vi "Main.vi"() -> ()   [LabVIEW 2017, in "Akwizycja.lvlib"]
doc: "This template is based from the Queued Message Handler design pattern and the Queued Message Handler Project Template that ships with LabVIEW 2014.\n\nThe main difference is that the Queue is private to this module and communication between modules is done via Broadcast and Request events.\n\nRequest events are wrapped via public API methods and are handled in the Event handler loop in this VI.\nAny module can register for Broadcast events sent by this module.\n\nThe Event Handling Loop generates messages based on user interface actions.\n\nThe Message Handling Loop processes messages generated by the Event Handling Loop, or by other messages. The messages are string values, so new messages can be added easily to the Message Cases case structure in the Message Handling Loop. Each message cluster can also provide an optional value for Message Data, which is a variant that can be converted to whatever message-specific data is required.\n_____\nBased on Delacor QMH Project Template 3.1.0.34."
uses:
  Akwizycja.lvlib
  <vilib>/Delacor/Delacor QMH/Libraries/Module Admin_class/Delacor_lib_QMH_Module Admin.lvclass
  Time Events cluster.ctl
  Time events enum.ctl
  Module Data--cluster.ctl
  Show Panel Argument--cluster.ctl
  Hide Panel Argument--cluster.ctl
  Stop Argument--cluster.ctl
  <vilib>/Delacor/Delacor QMH/Libraries/Module Admin_class/Delacor_lib_QMH_Module Admin.lvclass/Delacor_lib_QMH_Module Admin.ctl
  Read Slaves Argument--cluster.ctl
  <vilib>/Utility/miscctls.llb/LVPointTypeDef.ctl
  <vilib>/Delacor/Delacor QMH/Libraries/Module Admin_class/Delacor_lib_QMH_Get External Launch.vi
  <vilib>/Utility/error.llb/Error Cluster From Error Code.vi
  <vilib>/Delacor/Delacor QMH/Libraries/Message Queue_class/Delacor_lib_QMH_Enqueue Message (Single).vi
  <vilib>/ErrorRing/Error Ring.xnode
  <vilib>/Delacor/Delacor QMH/Libraries/Message Queue_class/Delacor_lib_QMH_Message Queue.lvclass
  <vilib>/Plasmionique/MB Master/MB_Master_Serial/MB_Master_Serial.lvclass
panel:
  out "error obsrany":errorcluster
  in  "log_avg_c":dbl
  in  "Time Events":T1
  in  "Registers 2":u16[][](array[numeric])
  out "read_slaves":bool
  out "Elapsed Time (s)":dbl
  out "stop_time":bool
  in  "Simulate MHL Error":bool
  in  "Simulate EHL Error":bool
  out "error out":errorcluster
  in  "Module Admin":refnum<class "Delacor_lib_QMH_Module Admin.lvclass">
  out "Status":string
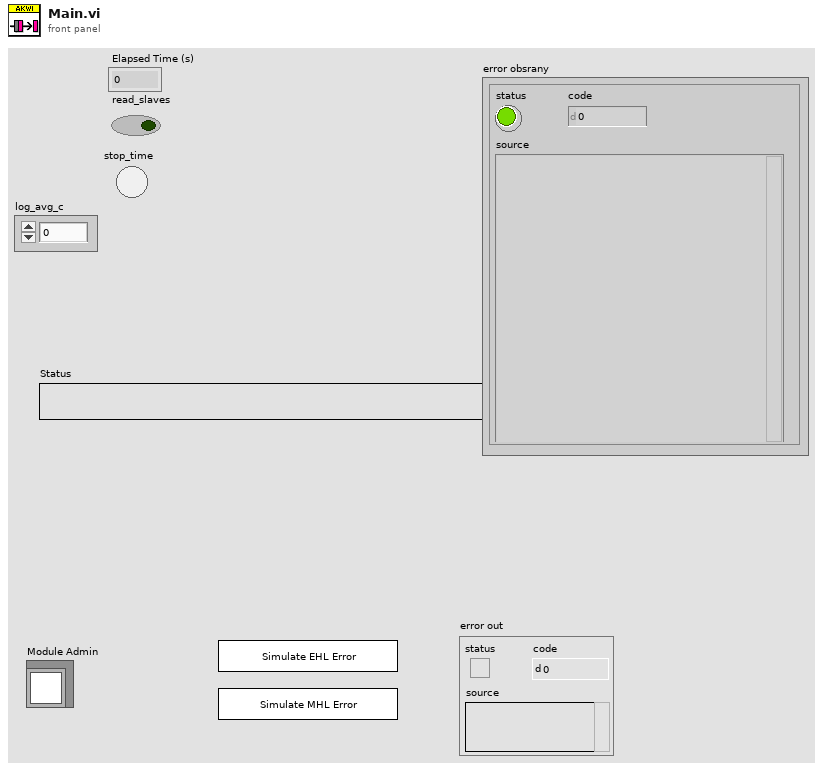
[diagram p1: front panel]
types:
  T1 = typedef "Time Events cluster.ctl" = cluster{"Read Slaves":refnum<user-event>, "Log Avg":refnum<user-event>}
  T2 = typedef "Time events enum.ctl" = enum16{"read_slaves", "log_avg"}
  T3 = typedef "Akwizycja.lvlib/Request Events--cluster.ctl" = cluster{"Stop Module":refnum<user-event>, "Show Panel":refnum<user-event>, "Hide Panel":refnum<user-event>, "Get Module Execution Status":refnum<user-event>, "Show Diagram":refnum<user-event>, "Read Slaves":refnum<user-event>}
  T4 = typedef "Akwizycja.lvlib/Module Data--cluster.ctl" = cluster{"Status":string}
  T5 = typedef "Akwizycja.lvlib/Show Panel Argument--cluster.ctl" = cluster{"Show Panel?":bool}
  T6 = typedef "Akwizycja.lvlib/Hide Panel Argument--cluster.ctl" = cluster{"Hide Panel?":bool}
  T7 = typedef "Akwizycja.lvlib/Stop Argument--cluster.ctl" = cluster{"Origin":string, "Exit via Stop Module Req?":bool, "Wait for Module to stop?":bool}
  T8 = typedef "Akwizycja.lvlib/Read Slaves Argument--cluster.ctl" = cluster{"Boolean":bool}
  T9 = typedef "LVPointTypeDef.ctl" = cluster{"Horizontal":i16, "Vertical":i16}
  T10 = enum32{"Invalid", "Standard", "Closed", "Hidden", "Minimized", "Maximized"}
  T11 = enum32{"invalid lock state", "Not Locked", "Locked (No Password)", "Password-protected"}
  T12 = cluster{"Fuel Flow":dbl[][][], "Init array":refnum<class "MB_Master_Serial.lvclass">[], "Array of temperatures":dbl[][][]}
  T13 = cluster{"Fuel Flow":dbl[][][], "Init array":refnum<class "MB_Master_Serial.lvclass">[], "Temps":dbl[][][]}
  T14 = cluster{"Combined Fuel Flows":dbl[][][], "Serial out":refnum<class "MB_Master_Serial.lvclass">[], "Combined Temps":dbl[][][]}
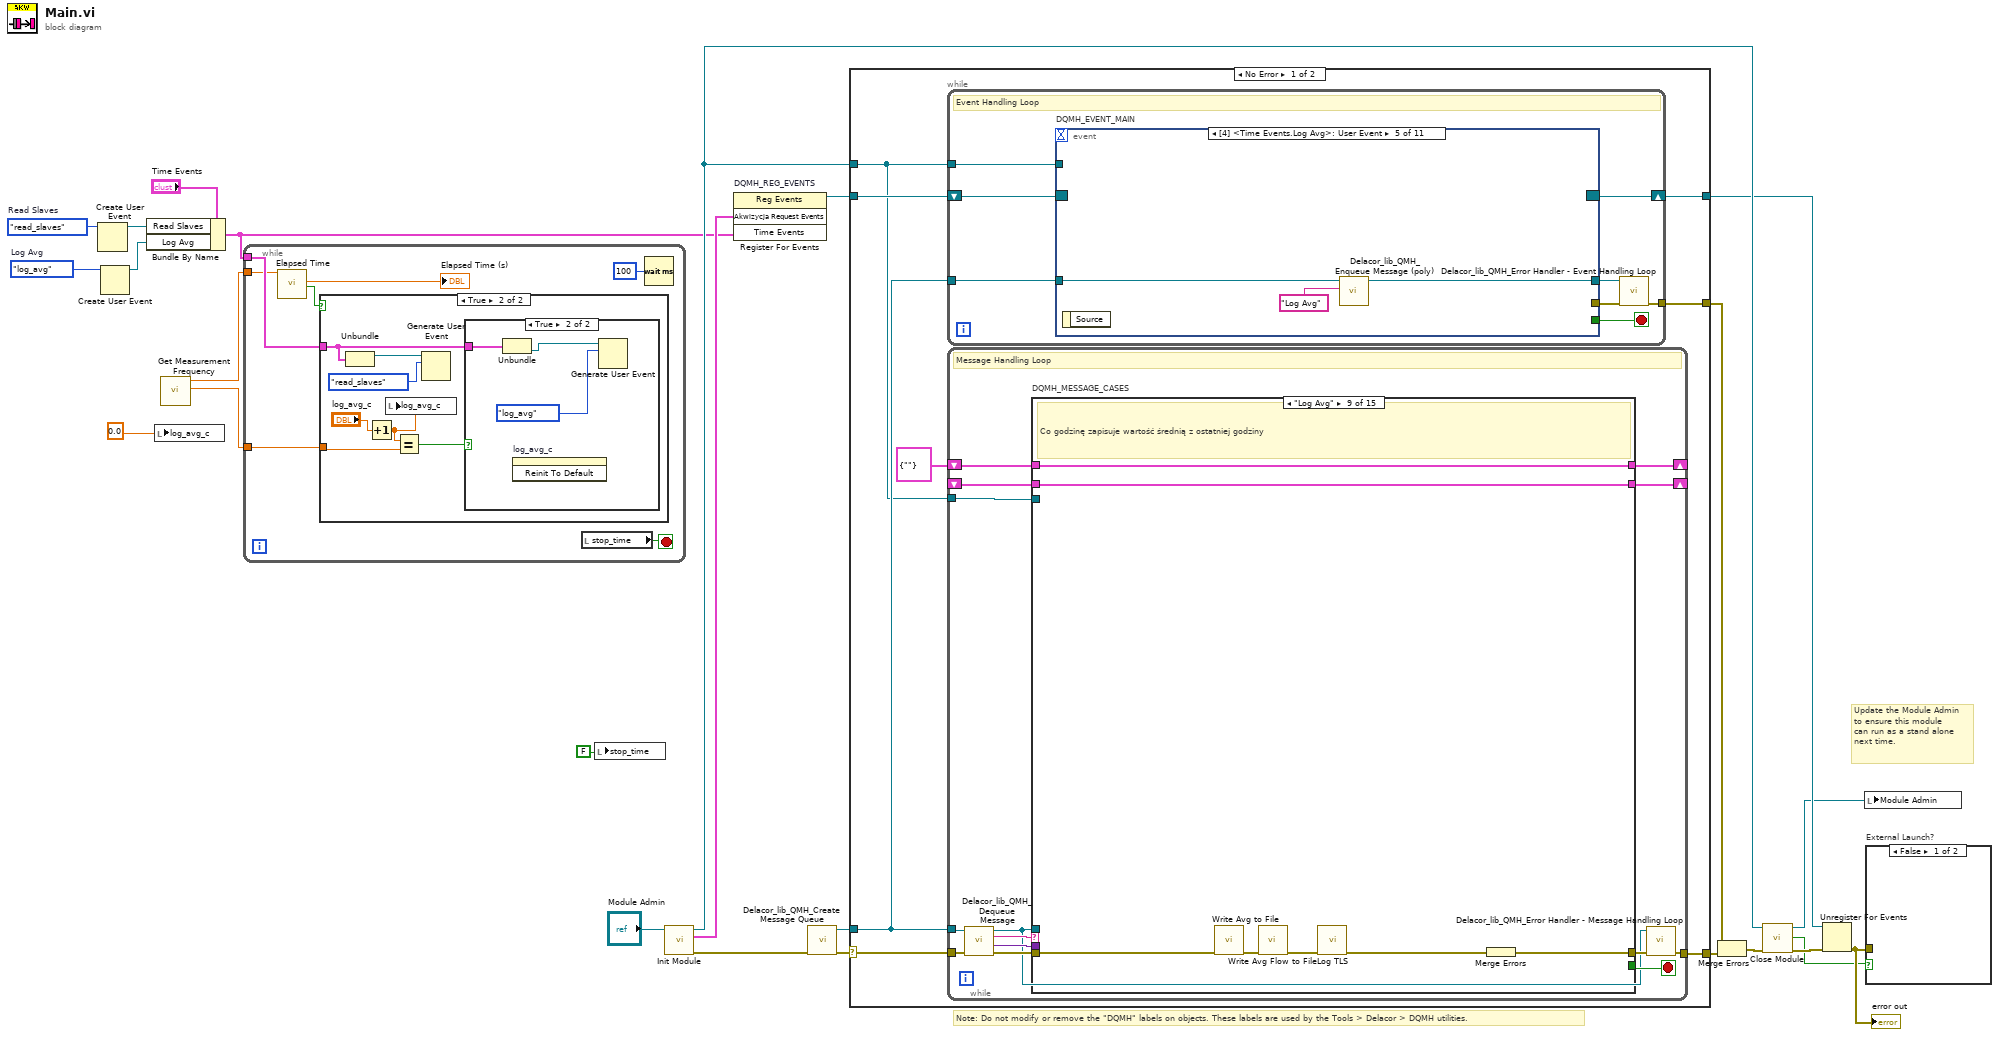
[diagram p0: block diagram]
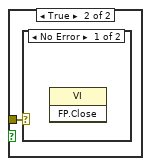
[diagram p4: hidden frame]
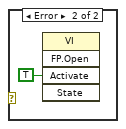
[diagram p5: hidden frame]
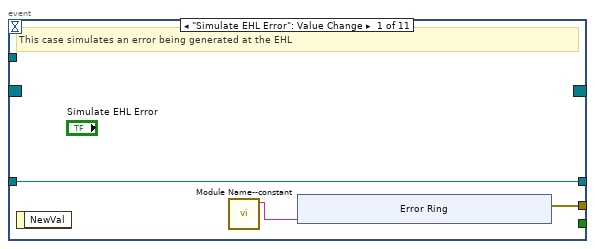
[diagram p6: hidden frame]
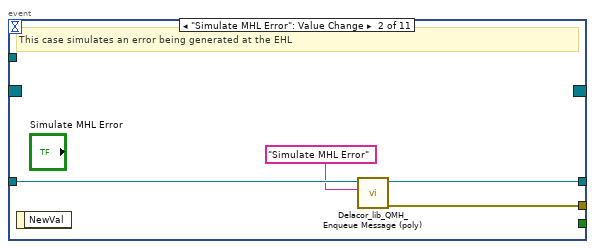
[diagram p7: hidden frame]
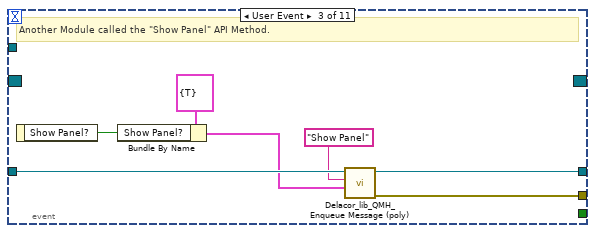
[diagram p8: hidden frame]
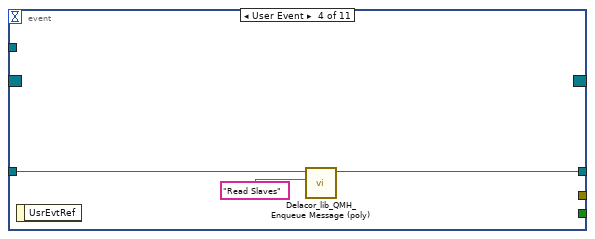
[diagram p9: hidden frame]
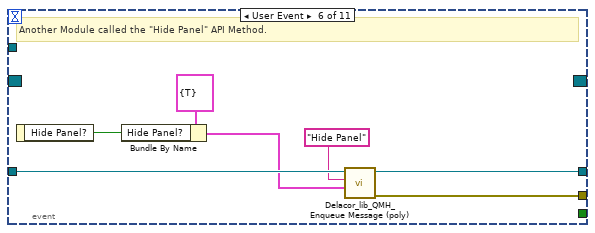
[diagram p10: hidden frame]
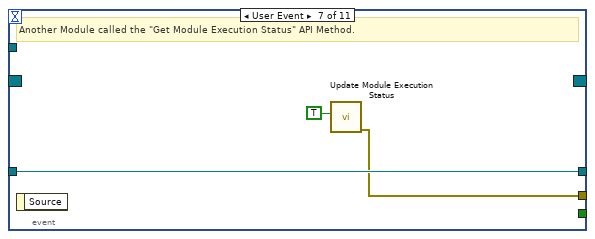
[diagram p11: hidden frame]
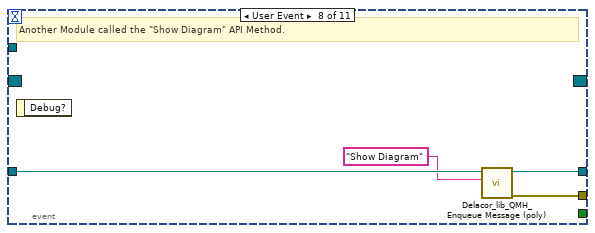
[diagram p12: hidden frame]
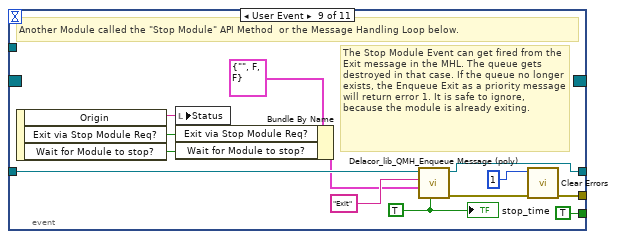
[diagram p13: hidden frame]
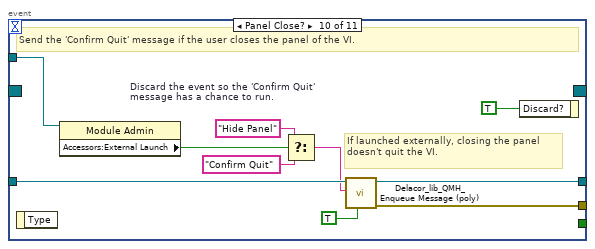
[diagram p14: hidden frame]
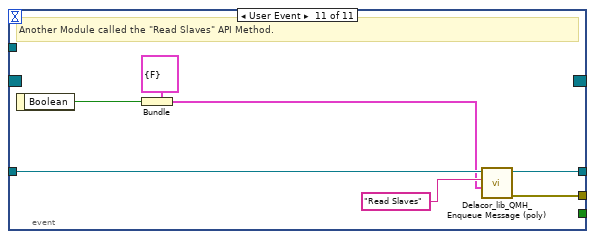
[diagram p15: hidden frame]
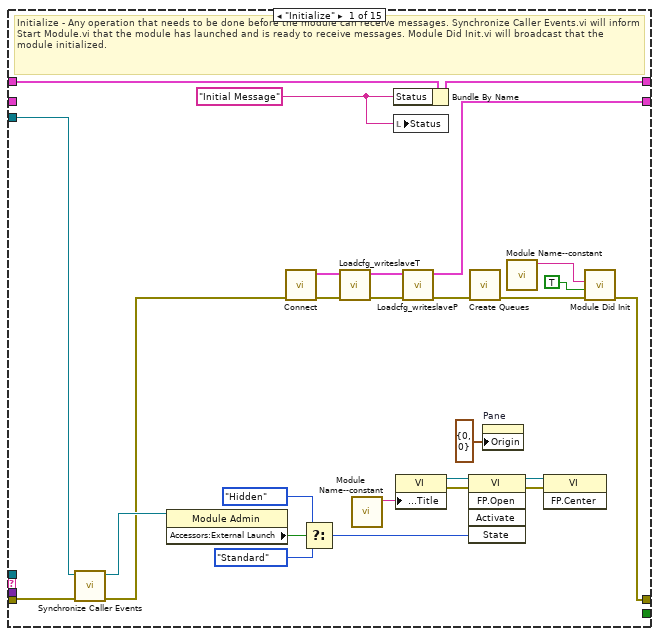
[diagram p16: hidden frame]
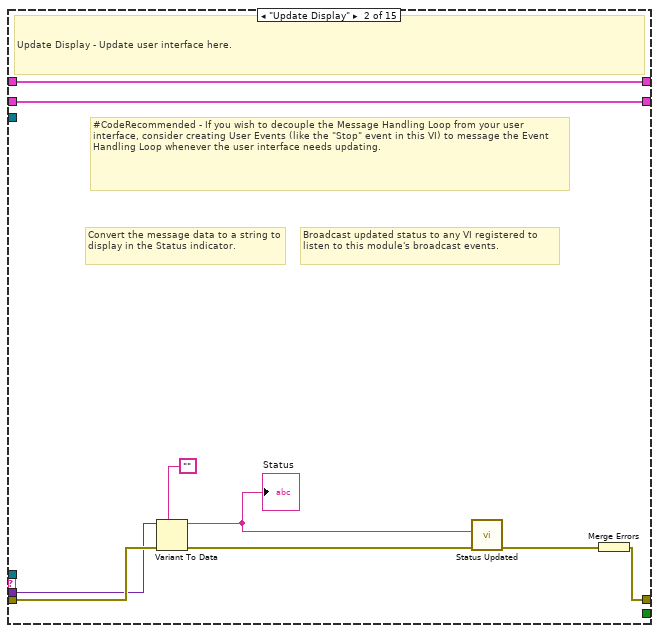
[diagram p17: hidden frame]
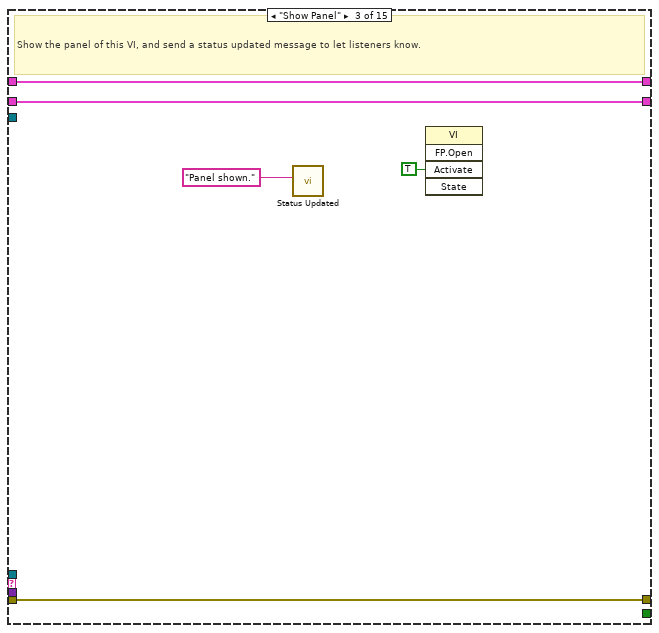
[diagram p18: hidden frame]
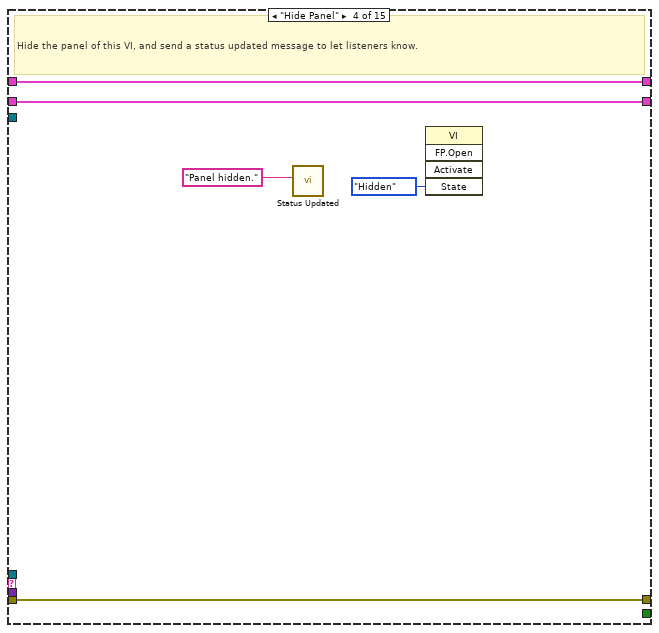
[diagram p19: hidden frame]
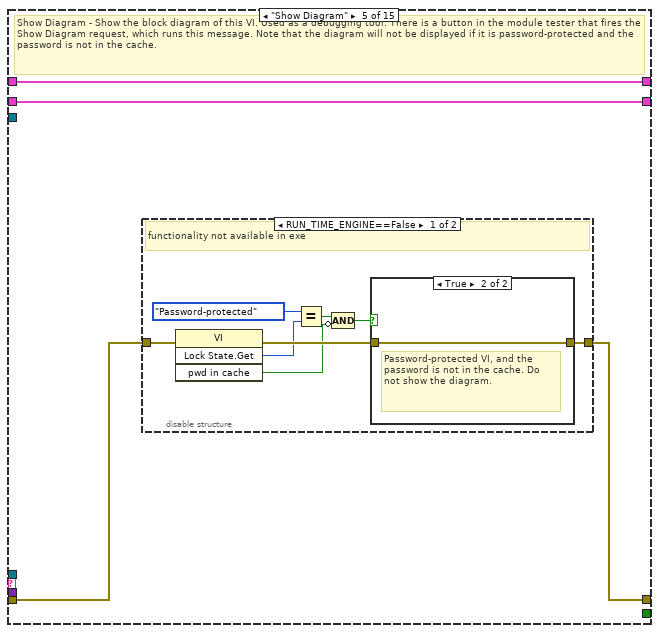
[diagram p20: hidden frame]
diagram:
  w5 = Time_events_enum."log_avg"  # Log Avg
  w9 = Time_events_enum."read_slaves"  # Read Slaves
  # "Note: Do not modify or remove the \"DQMH\" labels on objects. These labels are used by the Tools > Delacor > DQMH utilities."
  # "Update the Module Admin to ensure this module can run as a stand alone next time."
  n1 = Create User Event(user event datatype=w9) -> (user event=w8:refnum<user-event>)  [unwired: 1 in, 1 out]
  n2 = Create User Event(user event datatype=w5) -> (user event=w4:refnum<user-event>)  [unwired: 1 in, 1 out]
  n3 = Bundle By Name(cluster="Time Events", "Read Slaves"=w8, "Log Avg"=w4) -> (w6:T1)
  n4 = local write "log_avg_c"(0.0 ("log_avg_c")) -> ()
  n5 = call "Get Measurement Frequency.vi"() -> ("Measurments per hour"=w2:dbl, "Seconds"=w3:dbl)  [unwired: 10 in]
  n6 = while {
    tunnel: w6 -> [w28]
    tunnel: w3 -> [w27]
    tunnel: w2 -> [w26]
    stop <- w30 stop-if-true
    n7 = call "Elapsed Time"("Time Target (s)"=w27) -> ("Elapsed Time (s)"=→"Elapsed Time (s)":dbl, "Time has Elapsed"=w29:bool)  [unwired: 11 in, 6 out]
    n8 = case shown="True" w29 {
      tunnel: w28 -> [_ w33]
      tunnel: w26 -> [_ w35]
      frame False {
      }
      frame True {
        n9 = Unbundle(w33) -> ("Read Slaves"=w38:refnum<user-event>)  [unwired: 1 out]
        n10 = Increment(x="log_avg_c") -> (x+1=w36:dbl)
        n11 = local write "log_avg_c"(w36) -> ()
        n12 = Equal?(x=w36, y=w35) -> (x = y?=w34:bool)
        n13 = Generate User Event(user event=w38, event data cluster=Time_events_enum."read_slaves") -> ()  [unwired: 2 in, 2 out]
        n14 = case shown="True" w34 {
          tunnel: w33 -> [_ w40]
          frame False {
          }
          frame True {
            n15 = Unbundle(w40) -> ("Log Avg"=w41:refnum<user-event>)  [unwired: 1 out]
            n16 = invoke on="log_avg_c" class="DigNum (strict)" method="Reinit To Default"() -> ()  [unwired: 3 in, 3 out]
            n17 = Generate User Event(user event=w41, event data cluster=Time_events_enum."log_avg") -> ()  [unwired: 2 in, 2 out]
          }
        }
      }
    }
    n18 = local read "stop_time"() -> (w30:bool)
    n19 = Wait (ms)(milliseconds to wait=u32 100) -> ()  [unwired: 1 out]
  }
  n20 = local write "stop_time"(FALSE) -> ()
  n21 = call "Init Module.vi"("Singleton Module Admin in"="Module Admin") -> ("error out"=w23:errorcluster, "Akwizycja Request Events"=w20:T3, "Singleton Module Admin out"=w25:refnum<class "Delacor_lib_QMH_Module Admin.lvclass">)  [unwired: 8 in]
  n22 = register-events "DQMH_REG_EVENTS"(w20, w6) -> (reference out=w21:refnum<event-registration>)  [unwired: 2 in, 1 out]
  n23 = call <vilib>:"Delacor_lib_QMH_Create Message Queue.vi"("error in (no error)"=w23) -> ("error out"=w11:errorcluster, "Message Queue"=w19:refnum<class "Delacor_lib_QMH_Message Queue.lvclass">)  [unwired: 9 in]
  n24 = case shown="No Error" w11 {
    selector: w11 -> [w44 w378]
    tunnel: [w50 w378] -> w24
    tunnel: [w49 w383] -> w22
    tunnel: w21 -> [w47 w383]
    tunnel: w19 -> [w46 _]
    tunnel: [w45 _] -> w15
    tunnel: w25 -> [w43 w379]
    frame No Error {
      n25 = while {
        tunnel: w46 -> [w58]
        shift-right: [w56] -> w49
        shift-left: w47 -> [w57]
        tunnel: [w52] -> w45
        tunnel: w43 -> [w51]
        stop <- w54 stop-if-true
        # "Event Handling Loop"
        n26 = event "DQMH_EVENT_MAIN" shown="[4] <Time Events.Log Avg>: User Event" {
          selector: w57 -> [_ _ _ _ _ _ _ _ _ _ _]
          dyn-events: [_ _ _ _ _ _ _ _ _ _ _] -> w56
          timeout: _ -> [_ _ _ _ _ _ _ _ _ _ _]
          tunnel: [_ _ _ _ _ _ _ _ TRUE ("Discard?") _ _] -> w54
          tunnel: w58 -> [w61 w72 w79 w82 w84 w92 w95 w99 w110 w121 w129]
          tunnel: [w60 w69 w77 _ _ w90 w94 w96 w105 w120 w123] -> w55
          tunnel: [w61 w71 w78 w81 w83 w91 w95 w98 w109 w119 w128] -> w53
          tunnel: w51 -> [_ _ _ _ _ _ _ _ _ w115 _]
          event "Simulate EHL Error": Value Change {
            # "This case simulates an error being generated at the EHL"
            n27 = event-data() -> ()  [unwired: 1 in, 1 out]
            n28 = call "Module Name--constant.vi"() -> ("Module Name"=w59:string)  [unwired: 11 in]
            n29 = xnode "Error Ring"("parameter 0"=w59) -> ("error out"=w60:errorcluster)
          }
          event "Simulate MHL Error": Value Change {
            # "This case simulates an error being generated at the EHL"
            n30 = event-data() -> ()  [unwired: 1 in, 1 out]
            n31 = call-poly <vilib>:"Delacor_lib_QMH_Enqueue Message (poly).vi"("Message"="Simulate MHL Error", "Message Queue in"=w72) -> ("error out"=w69:errorcluster, "Message Queue out"=w71:refnum<class "Delacor_lib_QMH_Message Queue.lvclass">)  [unwired: 8 in]
          }
          event User Event {
            # "Another Module called the \"Show Panel\" API Method."
            n32 = event-data() -> ("Show Panel?"=w75:bool)  [unwired: 1 in]
            n33 = Bundle By Name(cluster=T5 {"Show Panel?"=TRUE} ("Show Panel Argument"), "Show Panel?"=w75) -> (w73:T5)
            n34 = call-poly <vilib>:"Delacor_lib_QMH_Enqueue Message (poly).vi"("Message Data"=w73, "Message"="Show Panel", "Message Queue in"=w79) -> ("error out"=w77:errorcluster, "Message Queue out"=w78:refnum<class "Delacor_lib_QMH_Message Queue.lvclass">)  [unwired: 7 in]
          }
          event User Event {
            n35 = event-data() -> ()  [unwired: 1 in, 1 out]
            n36 = call-poly <vilib>:"Delacor_lib_QMH_Enqueue Message (poly).vi"("Message"="Read Slaves", "Message Queue in"=w82) -> ("Message Queue out"=w81:refnum<class "Delacor_lib_QMH_Message Queue.lvclass">)  [unwired: 8 in, 1 out]
          }
          event User Event {
            n37 = event-data() -> ()  [unwired: 1 in, 1 out]
            n38 = call-poly <vilib>:"Delacor_lib_QMH_Enqueue Message (poly).vi"("Message"="Log Avg", "Message Queue in"=w84) -> ("Message Queue out"=w83:refnum<class "Delacor_lib_QMH_Message Queue.lvclass">)  [unwired: 8 in, 1 out]
          }
          event User Event {
            # "Another Module called the \"Hide Panel\" API Method."
            n39 = event-data() -> ("Hide Panel?"=w87:bool)  [unwired: 1 in]
            n40 = Bundle By Name(cluster=T6 {"Hide Panel?"=TRUE} ("Hide Panel Argument"), "Hide Panel?"=w87) -> (w86:T6)
            n41 = call-poly <vilib>:"Delacor_lib_QMH_Enqueue Message (poly).vi"("Message Data"=w86, "Message"="Hide Panel", "Message Queue in"=w92) -> ("error out"=w90:errorcluster, "Message Queue out"=w91:refnum<class "Delacor_lib_QMH_Message Queue.lvclass">)  [unwired: 7 in]
          }
          event User Event {
            # "Another Module called the \"Get Module Execution Status\" API Method."
            n42 = event-data() -> ()  [unwired: 1 in, 1 out]
            n43 = call "Update Module Execution Status.vi"("Running?"=TRUE) -> ("error out"=w94:errorcluster)  [unwired: 10 in]
          }
          event User Event {
            # "Another Module called the \"Show Diagram\" API Method."
            n44 = event-data() -> ()  [unwired: 1 in, 1 out]
            n45 = call-poly <vilib>:"Delacor_lib_QMH_Enqueue Message (poly).vi"("Message"="Show Diagram", "Message Queue in"=w99) -> ("error out"=w96:errorcluster, "Message Queue out"=w98:refnum<class "Delacor_lib_QMH_Message Queue.lvclass">)  [unwired: 8 in]
          }
          event User Event {
            w100 = TRUE ("Priority Message? (F)")
            # "The Stop Module Event can get fired from the Exit message in the MHL. The queue gets destroyed in that case. If the queue no longer exists, the Enqueue Exit as a priority message will return error 1. It is safe to ignore, because the module is already exiting."
            # "Another Module called the \"Stop Module\" API Method  or the Message Handling Loop below."
            n46 = event-data() -> ("Origin"=w108:string, "Exit via Stop Module Req?"=w103:bool, "Wait for Module to stop?"=w102:bool)  [unwired: 1 in]
            n47 = local write "Status"(w108) -> ()
            n48 = Bundle By Name(cluster=T7 {"Origin"="", "Exit via Stop Module Req?"=FALSE, "Wait for Module to stop?"=FALSE} ("Stop Argument"), "Exit via Stop Module Req?"=w103, "Wait for Module to stop?"=w102) -> (w101:T7)
            n49 = call-poly <vilib>:"Delacor_lib_QMH_Enqueue Message (poly).vi"("Priority Message? (F)"=w100, "Message Data"=w101, "Message"="Exit", "Message Queue in"=w110) -> ("error out"=w106:errorcluster, "Message Queue out"=w109:refnum<class "Delacor_lib_QMH_Message Queue.lvclass">)  [unwired: 6 in]
            n50 = call <vilib>:"Clear Errors.vi"("error in (no error)"=w106, "specific error code to clear (0: all)"=1) -> ("error out"=w105:errorcluster)  [unwired: 4 in, 1 out]
            "stop_time" <- w100
          }
          event Panel Close? {
            w122 = TRUE  # Discard the event so the 'Confirm Quit' message has a chance to run.
            # "If launched externally, closing the panel doesn't quit the VI."
            # "Send the 'Confirm Quit' message if the user closes the panel of the VI."
            n51 = event-data() -> ()  [unwired: 1 in, 1 out]
            n52 = property class="Module Admin"(reference=w115) -> ("Accessors:External Launch"=w114:bool)  [unwired: 1 in, 2 out]
            n53 = Select(t="Hide Panel" ("Message"), s=w114, f="Confirm Quit" ("Message")) -> (s? t:f=w116:string)
            n54 = call-poly <vilib>:"Delacor_lib_QMH_Enqueue Message (poly).vi"("Priority Message? (F)"=TRUE, "Message"=w116, "Message Queue in"=w121) -> ("error out"=w120:errorcluster, "Message Queue out"=w119:refnum<class "Delacor_lib_QMH_Message Queue.lvclass">)  [unwired: 7 in]
            n55 = event-data("Discard?"=w122) -> ()  [unwired: 1 in, 1 out]
          }
          event User Event {
            # "Another Module called the \"Read Slaves\" API Method."
            n56 = event-data() -> ("Boolean"=w124:bool)  [unwired: 1 in]
            n57 = Bundle(cluster=T8 {"Boolean"=FALSE} ("Read Slaves Argument"), "Boolean"=w124) -> (w125:T8)
            n58 = call-poly <vilib>:"Delacor_lib_QMH_Enqueue Message (poly).vi"("Message Data"=w125, "Message"="Read Slaves", "Message Queue in"=w129) -> ("error out"=w123:errorcluster, "Message Queue out"=w128:refnum<class "Delacor_lib_QMH_Message Queue.lvclass">)  [unwired: 7 in]
          }
        }
        n59 = call-dynamic "Delacor_lib_QMH_Error Handler - Event Handling Loop.vi"("error in (no error)"=w55, "Message Queue in"=w53) -> ("dup error in"=w52:errorcluster)  [unwired: 8 in, 1 out]
      }
      n60 = while {
        tunnel: w46 -> [w135]
        shift-right: [w141] -> _
        shift-left: T4 {"Status"=""} ("Data Cluster") -> [w142]
        tunnel: w44 -> [w139]
        tunnel: [w134] -> w50
        tunnel: w43 -> [w133]
        shift-right: [w132] -> _
        shift-left: _ -> [w131]
        stop <- w140 stop-if-true
        # "Message Handling Loop"
        n61 = call-dynamic "Delacor_lib_QMH_Dequeue Message.vi"("error in (no error)"=w139, "Message Queue in"=w135) -> ("error out"=w138:errorcluster, "Message Data"=w136:variant, "Message"=w137:string, "Message Queue out"=w130:refnum<class "Delacor_lib_QMH_Message Queue.lvclass">)  [unwired: 6 in]
        n62 = case "DQMH_MESSAGE_CASES" shown="\"Log Avg\"" w137 {
          selector: w137 -> [_ _ _ _ _ _ _ _ _ _ _ _ _ _ w365]
          tunnel: w130 -> [_ _ _ _ _ _ _ w239 _ _ _ w299 w331 w357 _]
          tunnel: w138 -> [w160 w177 w184 w186 w192 w208 w232 w238 w270 w277 w283 w303 w335 w359 _]
          tunnel: [w147 w178 w184 w186 w191 w214 w230 w241 w272 w275 w281 w294 w333 w354 w366] -> w143
          tunnel: w142 -> [w159 w179 w183 w189 w193 w228 w231 w242 w273 w276 w282 w302 w334 w356 w367]
          tunnel: [w158 w179 w183 w189 w193 w228 w231 w242 w273 w276 w282 w302 w334 w356 w367] -> w141
          tunnel: [_ _ _ _ _ _ _ _ _ _ _ _ _ w346 _] -> w140
          tunnel: w136 -> [_ w176 _ _ _ _ _ _ _ _ _ w301 _ w353 _]
          tunnel: w133 -> [w161 _ _ _ _ _ _ _ _ _ _ w298 _ w347 _]
          tunnel: [w144 w171 w180 w185 w190 w224 w229 w236 w271 w274 w278 w296 w328 w338 w363] -> w132
          tunnel: w131 -> [_ w171 w180 w185 w190 w225 w229 w240 w271 w274 w278 w296 w328 w338 w363]
          frame "Initialize" {
            w157 = "Initial Message" ("Initial Message")
            # "Initialize - Any operation that needs to be done before the module can receive messages. Synchronize Caller Events.vi will inform Start Module.vi that the module has launched and is ready to receive messages. Module Did Init.vi will broadcast that the module initialized."
            n63 = call "Synchronize Caller Events.vi"("error in (no error)"=w160, "Singleton Module Admin in"=w161) -> ("error out"=w148:errorcluster, "Singleton Module Admin out"=w156:refnum<class "Delacor_lib_QMH_Module Admin.lvclass">)  [unwired: 8 in]
            n64 = property class="Module Admin"(reference=w156) -> ("Accessors:External Launch"=w165:bool)  [unwired: 1 in, 2 out]
            n65 = call "Connect.vi"("error in"=w148) -> ("error out"=w153:errorcluster, "Data Cluster"=w146:T12)  [unwired: 9 in]
            n66 = Select(t=T10."Hidden" ("State"), s=w165, f=T10."Standard" ("State")) -> (s? t:f=w162:T10)
            n67 = call "Loadcfg_writeslaveT.vi"("error in"=w153, "Data Cluster in"=w146) -> ("error out"=w154:errorcluster, "Data Cluster out"=w145:T13)  [unwired: 8 in]
            n68 = call "Module Name--constant.vi"() -> ("Module Name"=w170:string)  [unwired: 11 in]
            n69 = Bundle By Name(cluster=w159, "Status"=w157) -> (w158:T4)
            n70 = local write "Status"(w157) -> ()
            n71 = property class="VI"("Front Panel.Title"=w170) -> (reference out=w168:refnum<vi>, error out=w169:errorcluster)  [unwired: 2 in]
            n72 = call "Loadcfg_writeslaveP.vi"("error in"=w154, "Data Cluster in"=w145) -> ("error out"=w150:errorcluster, "Data Cluster out"=w144:T13)  [unwired: 8 in]
            n73 = invoke class="VI" method="FP.Open"(reference=w168, error in=w169, "State"=w162) -> (reference out=w167:refnum<vi>, error out=w166:errorcluster)  [unwired: 2 in, 3 out]
            n74 = call "Create Queues.vi"("error in (no error)"=w150) -> ("error out"=w149:errorcluster)  [unwired: 10 in]
            n75 = property on="Pane" class="Pane"("Origin"=T9 {"Horizontal"=0, "Vertical"=0}) -> ()  [unwired: 2 in, 2 out]
            n76 = call "Module Name--constant.vi"() -> ("Module Name"=w152:string)  [unwired: 11 in]
            n77 = invoke class="VI" method="FP.Center"(reference=w167, error in=w166) -> ()  [unwired: 1 in, 3 out]
            n78 = call "Module Did Init.vi"("error in (no error)"=w149, "Initialized?"=TRUE, "Origin"=w152) -> ("error out"=w147:errorcluster)  [unwired: 8 in]
          }
          frame "Update Display" {
            # "Broadcast updated status to any VI registered to listen to this module's broadcast events."
            # "Convert the message data to a string to display in the Status indicator."
            # "#CodeRecommended - If you wish to decouple the Message Handling Loop from your user interface, consider creating User Events (like the \"Stop\" event in this VI) to message the Event Handling Loop whenever the user interface needs updating."
            # "Update Display - Update user interface here."
            n79 = Variant To Data(error in=w177, type="", Variant=w176) -> (data=w174:string, error out=w173:errorcluster)
            "Status" <- w174
            n80 = call "Status Updated.vi"("error in (no error)"=w173, "Status"=w174) -> ("error out"=w172:errorcluster)  [unwired: 9 in]
            n81 = Merge Errors(w172) -> (w178:errorcluster)
          }
          frame "Show Panel" {
            # "Show the panel of this VI, and send a status updated message to let listeners know."
            n82 = call "Status Updated.vi"("Status"="Panel shown." ("format string")) -> ()  [unwired: 10 in, 1 out]
            n83 = invoke class="VI" method="FP.Open"("Activate"=TRUE ("Activate?")) -> ()  [unwired: 4 in, 5 out]
          }
          frame "Hide Panel" {
            # "Hide the panel of this VI, and send a status updated message to let listeners know."
            n84 = call "Status Updated.vi"("Status"="Panel hidden." ("format string")) -> ()  [unwired: 10 in, 1 out]
            n85 = invoke class="VI" method="FP.Open"("State"=T10."Hidden") -> ()  [unwired: 4 in, 5 out]
          }
          frame "Show Diagram" {
            # "Show Diagram - Show the block diagram of this VI. Used as a debugging tool. There is a button in the module tester that fires the Show Diagram request, which runs this message. Note that the diagram will not be displayed if it is password-protected and the password is not in the cache."
            n86 = disable-structure shown="RUN_TIME_ENGINE==False" {
              disable-tunnel: [w201 w207] -> w191
              disable-tunnel: w192 -> [w200 w207]
              frame condition #0 (active) {
                # "functionality not available in exe"
                n87 = invoke class="VI" method="Lock State.Get"(error in=w200) -> (error out=w199:errorcluster, "Get Lock State"=w198:T11, "pwd in cache"=w195:bool)  [unwired: 3 in, 1 out]
                n88 = Equal?(x=T11."Password-protected", y=w198) -> (x = y?=w196:bool)
                n89 = Compound Arithmetic op=AND(w196, invert w195) -> (w194:bool)
                n90 = case shown="True" w194 {
                  tunnel: [w204 w206] -> w201
                  tunnel: w199 -> [w202 w206]
                  frame False {
                    n91 = property class="VI"(error in=w202, "BDWin.Open"=TRUE ("Block Diagram Window:Open")) -> (error out=w204:errorcluster)  [unwired: 1 in, 1 out]
                    n92 = call "Status Updated.vi"("Status"="Block Diagram shown." ("format string")) -> ()  [unwired: 10 in, 1 out]
                  }
                  frame True {
                    # "Password-protected VI, and the password is not in the cache. Do not show the diagram."
                  }
                }
              }
              frame condition #1 {
              }
            }
          }
          frame "Read Slaves" {
            # "Wywołanie modułu akwizycja do odczytania wartości z slave'ów"
            n93 = Unbundle(w225) -> ("Fuel Flow"=w218:dbl[][][], "Init array"=w211:refnum<class "MB_Master_Serial.lvclass">[], "Array of temperatures"=w219:dbl[][][])
            n94 = call "Read TLS.vi"("error in"=w208, "Serial in"=w211) -> ("error out"=w209:errorcluster, "Serial out"=w210:refnum<class "MB_Master_Serial.lvclass">[])  [unwired: 8 in]
            n95 = call "read_temp_registers.vi"("Serial sessions"=w210, "error in"=w209) -> ("Serial out"=w213:refnum<class "MB_Master_Serial.lvclass">[], "Array of temperatures"=w222:dbl[][], "error out"=w221:errorcluster)  [unwired: 6 in]
            n96 = call "Calculate Temp AVGs Send Temp.vi"("error in"=w221, "New Temps"=w222, "Old Temps"=w219) -> ("error out"=w215:errorcluster, "Combined Temps"=w223:dbl[][][])  [unwired: 7 in]
            n97 = call "Read Fuel.vi"("error in"=w215, "Serial sessions"=w213) -> ("error out"=w220:errorcluster, "Serial out"=w212:refnum<class "MB_Master_Serial.lvclass">[], "Fuel Flows"=w217:dbl[][])  [unwired: 7 in]
            n98 = local read "read_slaves"() -> (w227:bool)
            n99 = call "Calculate Fuel AVGs Send Fuel.vi"("error in"=w220, "Old Fuel Flows"=w218, "New Fuel Flows"=w217) -> ("error out"=w214:errorcluster, "Combined Fuel Flows"=w216:dbl[][][])  [unwired: 7 in]
            n100 = Not(x=w227) -> (.not. x?=→"read_slaves":bool)
            n101 = Bundle("Combined Fuel Flows"=w216, "Serial out"=w212, "Combined Temps"=w223) -> (w224:T14)  [unwired: 1 in]
          }
          frame "---Copy This Frame---" {
            # "Duplicate this frame when creating new messages.  Change this comment in the duplicated frame to describe this message."
            n102 = Merge Errors(w232) -> (w230:errorcluster)
          }
          frame "Restart" {
            # "Duplicate this frame when creating new messages.  Change this comment in the duplicated frame to describe this message."
            n103 = flat-sequence {
              tunnel: w240 -> [w245]
              tunnel: w239 -> [w247]
              tunnel: w238 -> [w246]
              tunnel: [w245] -> w237
              tunnel: [w244] -> w235
              tunnel: [w243] -> w234
              tunnel: w237 -> [w257]
              tunnel: [w256] -> w236
              tunnel: w235 -> [w255]
              tunnel: w234 -> [w254]
              tunnel: [w253] -> w233
              frame #0 {
                n104 = Unbundle(w245) -> ("Init array"=w248:refnum<class "MB_Master_Serial.lvclass">[])  [unwired: 2 out]
                n105 = Array Size(array=w248) -> (size(s)=w249:i32)
                n106 = call-dynamic "Delacor_lib_QMH_Flush Messages.vi"("error in (no error)"=w246, "Message Queue in"=w247) -> ("error out"=w243:errorcluster, "Message Queue out"=w244:refnum<class "Delacor_lib_QMH_Message Queue.lvclass">)  [unwired: 6 in, 2 out]
                n107 = for {
                  N: w249 -> [_]
                  tunnel: w248 -> [w252]
                  i -> [w251]
                  n108 = Index Array(array=w252, index=w251) -> (element=w250:refnum<class "MB_Master_Serial.lvclass">)
                  n109 = call-dynamic "Close Session.vi"("MB_Serial session"=w250) -> ()  [unwired: 10 in, 1 out]
                }
              }
              frame #1 {
                n110 = call "Device Restart on Error.vi"() -> ("Restarted?"=w258:bool)  [unwired: 2 in]
                n111 = case shown="True" w258 {
                  tunnel: w257 -> [w263 _]
                  tunnel: [w263 w266] -> w256
                  tunnel: w255 -> [w262 _]
                  tunnel: w254 -> [w261 w265]
                  tunnel: [w259 w264] -> w253
                  frame False {
                    n112 = call-poly <vilib>:"Delacor_lib_QMH_Enqueue Message (poly).vi"("error in (no error)"=w261, "Message"="Exit", "Message Queue in"=w262) -> ("error out"=w259:errorcluster)  [unwired: 7 in, 1 out]
                  }
                  frame True {
                    n113 = call "Connect.vi"("error in"=w265) -> ("error out"=w264:errorcluster, "Data Cluster"=w266:T12)  [unwired: 9 in]
                  }
                }
              }
            }
            n114 = Merge Errors(w233) -> (w241:errorcluster)
          }
          frame "Log Avg" {
            # "Co godzinę zapisuje wartość średnią z ostatniej godziny"
            n115 = call "Write Avg to File.vi"("error in"=w270) -> ("error out"=w269:errorcluster)  [unwired: 10 in]
            n116 = call "Write Avg Flow to File.vi"("error in"=w269) -> ("error out"=w268:errorcluster)  [unwired: 10 in]
            n117 = call "Log TLS.vi"("error in"=w268) -> ("error out"=w267:errorcluster)  [unwired: 10 in]
            n118 = Merge Errors(w267) -> (w272:errorcluster)
          }
          frame "--- Exit and Error Handling---" {
            # "Separator - The following cases handle errors and exit messages."
            n119 = Merge Errors(w277) -> (w275:errorcluster)
          }
          frame "Simulate MHL Error" {
            # "Simulate an error occurring at the MHL"
            n120 = call "Module Name--constant.vi"() -> ("Module Name"=w280:string)  [unwired: 11 in]
            n121 = xnode "Error Ring"("parameter 0"=w280) -> ("error out"=w279:errorcluster)
            n122 = Merge Errors(w283, w279) -> (w281:errorcluster)
          }
          frame "Error" {
            # "#CodeRecommended - If you ever change the name of this \"Error\" message, you'll need to update the name in the Check Loop Error.vi as well."
            # "#CodeRecommended - If the module is running in standalone mode (External Launch = FALSE), this code will pop up an error dialog and call the 'Exit' message if an error occurs. Add more fine-grained error handling here."
            # "Error - Check the error message data and respond accordingly. This message is sent by the \"Error Handler\" VIs at the end of each loop in this application."
            n123 = property class="Module Admin"(reference=w298) -> ("Accessors:External Launch"=w297:bool)  [unwired: 1 in, 2 out]
            n124 = Variant To Data(error in=w303, type=errorcluster {"status"=FALSE, "code"=0, "source"=""} ("error constant"), Variant=w301) -> (data=w292:errorcluster, error out=w295:errorcluster)
            "error obsrany" <- w292
            n125 = Unbundle By Name(w292) -> ("code"=w291:i32)
            n126 = call "Error Reported.vi"("Error"=w292) -> ()  [unwired: 10 in, 1 out]
            n127 = case shown="403483" w291 {
              selector: w291 -> [_ w313 w318 w323]
              tunnel: w299 -> [w307 w316 w320 w325]
              tunnel: w297 -> [w306 _ _ _]
              tunnel: [w305 w314 w319 w324] -> w293
              tunnel: w292 -> [w304 _ _ _]
              frame 0, Default {
                n128 = case shown="True" w306 {
                  tunnel: [w312 _] -> w305
                  tunnel: w307 -> [w311 _]
                  tunnel: w304 -> [w308 _]
                  frame False {
                    # "If the module is running standalone, then pop up an error dialog and call the \"Exit\" message."
                    n129 = call <vilib>:"Simple Error Handler.vi"("error in (no error)"=w308) -> ()  [unwired: 4 in, 5 out]
                    n130 = call-poly <vilib>:"Delacor_lib_QMH_Enqueue Message (poly).vi"("Priority Message? (F)"=TRUE, "Message"="Exit", "Message Queue in"=w311) -> ("error out"=w312:errorcluster)  [unwired: 7 in, 1 out]
                  }
                  frame True {
                    # "If the module was launched externally, calling the Error Reported broadcast VI is the only action performed by the \"Error\" message. The module's caller can then process the error appropriately."
                  }
                }
              }
              frame -1073807339 {
                n131 = Number To Decimal String(number=w313) -> ()  [unwired: 1 in, 1 out]
                n132 = call-poly <vilib>:"Delacor_lib_QMH_Enqueue Message (poly).vi"("Priority Message? (F)"=TRUE, "Message"="Restart", "Message Queue in"=w316) -> ("error out"=w314:errorcluster)  [unwired: 7 in, 1 out]
              }
              frame -1073807360 {
                n133 = Number To Decimal String(number=w318) -> ()  [unwired: 1 in, 1 out]
                n134 = call-poly <vilib>:"Delacor_lib_QMH_Enqueue Message (poly).vi"("Priority Message? (F)"=TRUE, "Message"="Restart", "Message Queue in"=w320) -> ("error out"=w319:errorcluster)  [unwired: 7 in, 1 out]
              }
              frame 403483 {
                n135 = Number To Decimal String(number=w323) -> ()  [unwired: 1 in, 1 out]
                n136 = call-poly <vilib>:"Delacor_lib_QMH_Enqueue Message (poly).vi"("Priority Message? (F)"=TRUE, "Message"="Restart", "Message Queue in"=w325) -> ("error out"=w324:errorcluster)  [unwired: 7 in, 1 out]
              }
            }
            n137 = Merge Errors(w293, w295) -> (w294:errorcluster)
            n138 = local write "error out"(w294) -> ()
          }
          frame "Confirm Quit" {
            # "#CodeNeeded - If you want to provide an \"Are you sure\" dialog (or some other notification) before the application exits, place that code here. This message is typically sent from a Panel Close? event."
            # "Confirm Quit - Message that can confirm whether or not the user wants to exit the application."
            n139 = call-poly <vilib>:"Delacor_lib_QMH_Enqueue Message (poly).vi"("Priority Message? (F)"=TRUE, "error in (no error)"=w335, "Message"="Exit", "Message Queue in"=w331) -> ("error out"=w332:errorcluster)  [unwired: 6 in, 1 out]
            n140 = Merge Errors(w332) -> (w333:errorcluster)
          }
          frame "Exit" {
            w351 = 91  # 91: not all Exit messages will have an argument
            w346 = TRUE  # Stop the VI
            # "Release the message queue reference"
            # "Exit - Exit the application."
            n141 = Variant To Data(error in=w359, type=T7 {"Origin"="", "Exit via Stop Module Req?"=FALSE, "Wait for Module to stop?"=FALSE} ("Stop Argument"), Variant=w353) -> (data=w349:T7, error out=w352:errorcluster)
            n142 = call <vilib>:"Clear Errors.vi"("error in (no error)"=w352, "specific error code to clear (0: all)"=w351) -> ("error out"=w358:errorcluster)  [unwired: 4 in, 1 out]
            n143 = control-ref of="This VI"() -> (w348:refnum<vi>)
            n144 = call "Handle Exit.vi"("Stop Argument"=w349, "Admin in"=w347, "VI reference"=w348) -> ("error out"=w345:errorcluster)  [unwired: 7 in, 1 out]
            n145 = Unbundle(w338) -> ("Init array"=w337:refnum<class "MB_Master_Serial.lvclass">[])  [unwired: 2 out]
            n146 = call-dynamic "Delacor_lib_QMH_Release Message Queue.vi"("error in (no error)"=w358, "Message Queue"=w357) -> ("error out"=w355:errorcluster)  [unwired: 9 in]
            n147 = Array Size(array=w337) -> (size(s)=w339:i32)
            n148 = Obtain Queue(name (unnamed)="temp_q", element data type="Registers 2") -> (queue out=w342:refnum<queue>, error out=w341:errorcluster)  [unwired: 3 in, 1 out]
            n149 = for {
              N: w339 -> [_]
              tunnel: w337 -> [w362]
              i -> [w361]
              n150 = Index Array(array=w362, index=w361) -> (element=w360:refnum<class "MB_Master_Serial.lvclass">)
              n151 = call-dynamic "Close Session.vi"("MB_Serial session"=w360) -> ()  [unwired: 10 in, 1 out]
            }
            n152 = Release Queue(queue=w342, force destroy? (F)=TRUE, error in (no error)=w341) -> (error out=w336:errorcluster)  [unwired: 2 out]
            n153 = Merge Errors(w336, w345, w355) -> (w354:errorcluster)
          }
          frame Default {
            # "'Default' case only runs if there is a message that isn't defined in any of the other cases.  Output a programming error."
            n154 = call "Module Name--constant.vi"() -> ("Module Name"=w364:string)  [unwired: 11 in]
            n155 = xnode "Error Ring"("parameter 0"=w365, "parameter 1"=w364) -> ("error out"=w366:errorcluster)
          }
        }
        n156 = call-dynamic "Delacor_lib_QMH_Error Handler - Message Handling Loop.vi"("error in (no error)"=w143, "Message Queue in"=w130) -> ("dup error in"=w134:errorcluster)  [unwired: 8 in, 1 out]
      }
    }
    frame Error {
      # "Synchronize Caller Events.vi will inform Start Module.vi that the module has launched and will let the code calling Start Module.vi register for broadcasts and would permit the caller receive the broadcast that an error occurred at launch time."
      n157 = call "Synchronize Caller Events.vi"("Singleton Module Admin in"=w379) -> ("error out"=w376:errorcluster)  [unwired: 9 in, 1 out]
      n158 = call "Module Name--constant.vi"() -> ("Module Name"=w382:string)  [unwired: 11 in]
      n159 = Format Into String(format string="An error occurred during initialization. %s is no longer running.", w382) -> (resulting string=w380:string)  [unwired: 2 in, 1 out]
      n160 = Merge Errors(w378, w376) -> (w377:errorcluster)
      n161 = call "Error Reported.vi"("Additional Information"=w380, "Error"=w377) -> ()  [unwired: 9 in, 1 out]
    }
  }
  n162 = Merge Errors(w15, w24) -> (w14:errorcluster)
  n163 = call "Close Module.vi"("error in (no error)"=w14, "Module Admin in"=w25) -> ("error out"=w17:errorcluster, "External Launch"=w12:bool, "Module Admin out"=w16:refnum<class "Delacor_lib_QMH_Module Admin.lvclass">)  [unwired: 7 in]
  n164 = Unregister For Events(event registration refnum=w22, error in=w17) -> (error out=w13:errorcluster)
  "error out" <- w13
  n165 = local write "Module Admin"(w16) -> ()
  n166 = case "External Launch?" shown="False" w12 {
    tunnel: w13 -> [_ w384]
    frame False {
    }
    frame True {
      n167 = case shown="No Error" w384 {
        frame No Error {
          n168 = invoke class="VI" method="FP.Close"() -> ()  [unwired: 3 in, 3 out]
        }
        frame Error {
          n169 = invoke class="VI" method="FP.Open"("Activate"=TRUE ("Activate?")) -> ()  [unwired: 4 in, 5 out]
        }
      }
    }
  }
